vi "AD DA test.vi"() -> ()   [LabVIEW 2010]
uses:
  <vilib>/DAQmx/read.llb/DAQmx Read (Analog DBL 1Chan 1Samp).vi
  <vilib>/DAQmx/write.llb/DAQmx Write (Analog DBL 1Chan 1Samp).vi
  <vilib>/DAQmx/create/channels.llb/DAQmx Create Channel (AI-Voltage-Basic).vi
  <vilib>/DAQmx/configure/timing.llb/DAQmx Timing (Sample Clock).vi
  <vilib>/DAQmx/create/channels.llb/DAQmx Create Channel (AO-Voltage-Basic).vi
  <vilib>/daqmx/miscellaneous.llb/DAQmx Fill In Error Info.vi
panel:
  in  "sample mode":i32(ring)=12522 items=["Finite Samples"=10178, "Continuous Samples"=10123, "Hardware Timed Single Point"=12522]
  out "Waveform Chart":dbl(graph)
  in  "DAQ input":tag
  in  "DAQ output":tag
  out "message":string=" INSTRUCTIONS:\r\rNormal Use:  When using subVIs that incorporate the error in/error out (or error I/O) structure, place this handler where you want to inform the user of an error, typically at the end of the I/O data path, as the last action of the program.  If the error in error? is ERROR, the handler creates a message describing the error and its source.  If the type of dialog = 1 (default), the message is displayed to the user, who can only acknowedge it.  If the type = 2, the user can acknowledge the message or abort execution; aborting a program with active I/O is not recommended.  If the type = 0, no message is displayed; this is used to process the error programmatically, and the error out cluster elements are wired to individual terminals for that reason.  \r\rOther Use:\n\r\nlocal testing.  To test the error code of a subVI or function that does not have the error I/O structure, you can wire its error code and a source string to the local error code and error source inputs.  If error in error? indicates no error and error code is not equal to 0, the local code and source are substituted for the error in values, and error? is set TRUE (ERROR)."
  in  "取樣頻率":dbl=100000.0 min=1.0 max=2000000.0 step=1.0
  in  "stop":bool
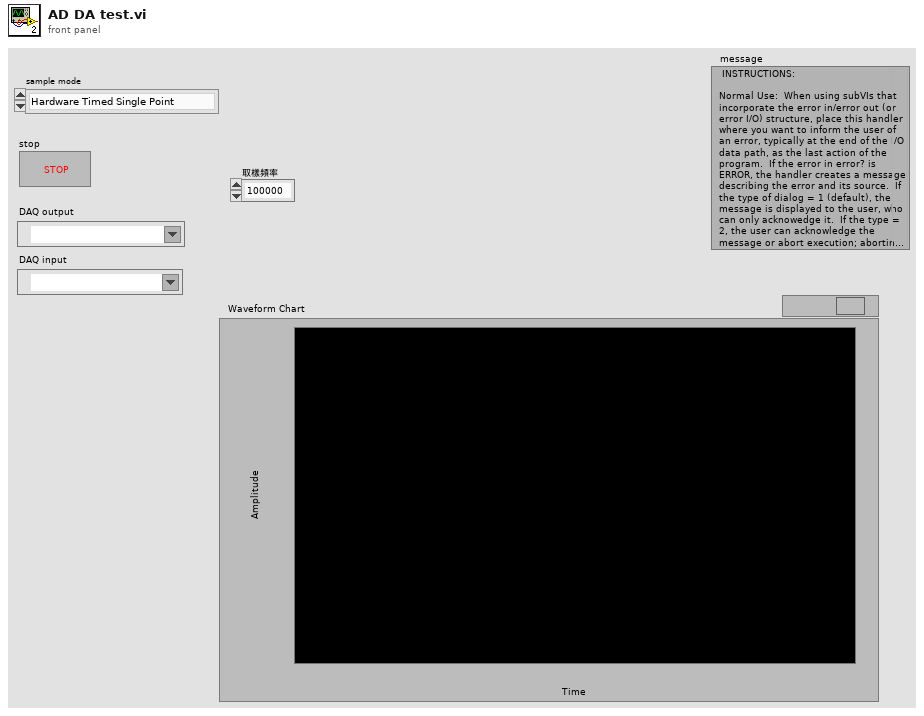
[diagram p1: front panel]
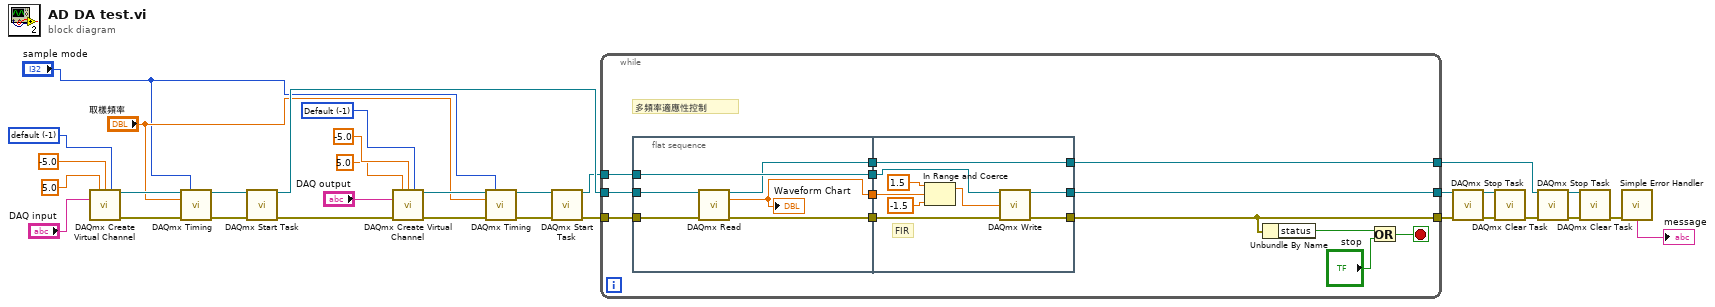
[diagram p0: block diagram]
diagram:
  w26 = -1 items=["Default"=-1, "RSE"=10083, "Differential"=10106, "Pseudodifferential"=12529] ("output terminal configuration")
  w25 = -1 items=["default"=-1, "RSE"=10083, "NRSE"=10078, "Differential"=10106, "Pseudodifferential"=12529] ("input terminal configuration")
  n1 = call-poly <vilib>:"DAQmx Create Virtual Channel.vi"("maximum value"=5.0, "minimum value"=-5.0, "input terminal configuration"=w25, "physical channels"="DAQ input") -> ("task out"=w17:refnum<k21>, "error out"=w20:errorcluster)  [unwired: 10 in]
  n2 = call-poly <vilib>:"DAQmx Timing.vi"("task/channels in"=w17, "sample mode"="sample mode", "rate"="取樣頻率", "error in"=w20) -> ("task out"=w18:refnum<k21>, "error out"=w19:errorcluster)  [unwired: 10 in]
  n3 = call <vilib>:"DAQmx Start Task.vi"("task/channels in"=w18, "error in"=w19) -> ("task out"=w16:refnum<k21>, "error out"=w31:errorcluster)  [unwired: 12 in]
  n4 = call-poly <vilib>:"DAQmx Create Virtual Channel.vi"("maximum value"=5.0, "minimum value"=-5.0, "output terminal configuration"=w26, "physical channels"="DAQ output", "error in"=w31) -> ("task out"=w24:refnum<k21>, "error out"=w21:errorcluster)  [unwired: 9 in]
  n5 = call-poly <vilib>:"DAQmx Timing.vi"("task/channels in"=w24, "sample mode"="sample mode", "rate"="取樣頻率", "error in"=w21) -> ("task out"=w23:refnum<k21>, "error out"=w22:errorcluster)  [unwired: 10 in]
  n6 = call <vilib>:"DAQmx Start Task.vi"("task/channels in"=w23, "error in"=w22) -> ("task out"=w14:refnum<k21>, "error out"=w15:errorcluster)  [unwired: 12 in]
  n7 = while {
    tunnel: w16 -> [w45]
    tunnel: w15 -> [w44]
    tunnel: w14 -> [w43]
    tunnel: [w42] -> w8
    tunnel: [w38] -> w7
    tunnel: [w41] -> w6
    stop <- w40 stop-if-true
    # "多頻率適應性控制"
    n8 = flat-sequence {
      tunnel: [w46] -> w36
      tunnel: [w49] -> w35
      tunnel: w45 -> [w51]
      tunnel: w44 -> [w50]
      tunnel: w43 -> [w48]
      tunnel: [w48] -> w34
      tunnel: [w47] -> w33
      tunnel: w35 -> [w59]
      tunnel: w36 -> [w52]
      tunnel: w34 -> [w60]
      tunnel: w33 -> [w56]
      tunnel: [w58] -> w42
      tunnel: [w57] -> w38
      tunnel: [w56] -> w41
      frame #0 {
        n9 = call-poly <vilib>:"DAQmx Read.vi"("task/channels in"=w51, "error in"=w50) -> ("task out"=w47:refnum<k21>, "data"=w46:dbl, "error out"=w49:errorcluster)  [unwired: 11 in]
        "Waveform Chart" <- w46
      }
      frame #1 {
        # "FIR"
        n10 = In Range and Coerce(upper limit=1.5, x=w52, lower limit=-1.5) -> (coerced(x)=w55:dbl)  [unwired: 1 out]
        n11 = call-poly <vilib>:"DAQmx Write.vi"("task/channels in"=w60, "data"=w55, "error in"=w59) -> ("task out"=w58:refnum<k21>, "error out"=w57:errorcluster)  [unwired: 10 in, 1 out]
      }
    }
    n12 = Unbundle By Name(w38) -> ("status"=w37:bool)
    n13 = Or(x=w37, y="stop") -> (x .or. y?=w40:bool)
  }
  n14 = call <vilib>:"DAQmx Stop Task.vi"("task/channels in"=w8, "error in"=w7) -> ("task out"=w9:refnum<k21>, "error out"=w10:errorcluster)  [unwired: 12 in]
  n15 = call <vilib>:"DAQmx Clear Task.vi"("task in"=w9, "error in"=w10) -> ("error out"=w13:errorcluster)  [unwired: 13 in]
  n16 = call <vilib>:"DAQmx Stop Task.vi"("task/channels in"=w6, "error in"=w13) -> ("task out"=w12:refnum<k21>, "error out"=w11:errorcluster)  [unwired: 12 in]
  n17 = call <vilib>:"DAQmx Clear Task.vi"("task in"=w12, "error in"=w11) -> ("error out"=w5:errorcluster)  [unwired: 13 in]
  n18 = call <vilib>:"Simple Error Handler.vi"("error in (no error)"=w5) -> ("message"=→"message":string)  [unwired: 4 in, 4 out]
